vi "Limit_Lookup.vi"(8 "all rows":string[][](array[string]), 11 "step name":string) -> (7 "found?":bool, 9 "high":dbl, 10 "low":dbl)   [LabVIEW 2026]
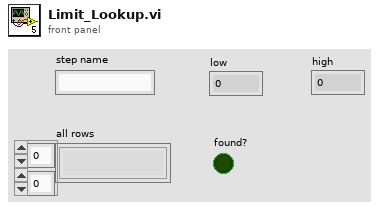
[diagram p1: front panel]
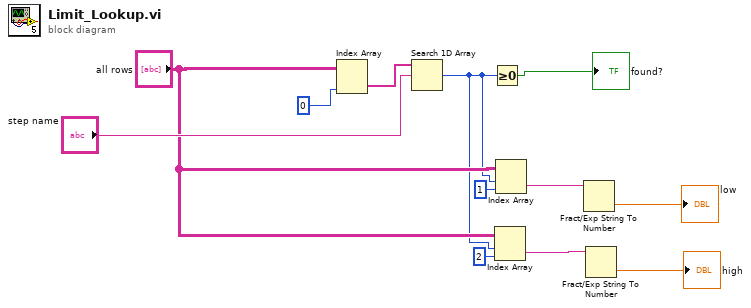
[diagram p0: block diagram]
diagram:
  n1 = Index Array(array="all rows", index (col)=0 ("index (row)")) -> (element=w11:string[])  [unwired: 1 in]
  n2 = Search 1D Array(1D array=w11, element="step name") -> (index of element=w5:i32)  [unwired: 1 in]
  n3 = Greater Or Equal To 0?(x=w5) -> (x >= 0?=→"found?":bool)
  n4 = Index Array(array="all rows", index (row)=w5, index (col)=2 ("disabled index (col)")) -> (element=w3:string)
  n5 = Index Array(array="all rows", index (row)=w5, index (col)=1 ("disabled index (col)")) -> (element=w4:string)
  n6 = Fract/Exp String To Number(string=w4) -> (number=→"low":dbl)  [unwired: 3 in, 1 out]
  n7 = Fract/Exp String To Number(string=w3) -> (number=→"high":dbl)  [unwired: 3 in, 1 out]
